vi "NI VeriStand - Get Custom Device Driver.vi"(8 "error in (no error)":errorcluster, 11 "Device Ref in":T4 format="%.0x") -> (0 "error out":errorcluster, 1 "Driver VI Path (Host)":T1, 2 "Driver VI Path (RT)":path, 3 "Device Ref out":T4 format="%.0x", 5 "Executon mode":T3)   [LabVIEW 2020, in "Custom Device Offline API.lvlib"]
uses:
  <vilib>/NI VeriStand/Custom Device Offline API/Custom Device Offline API.lvlib
  <vilib>/NI VeriStand/Custom Device API/Custom Device Item Ref.ctl
  <vilib>/NI VeriStand/Custom Device API/Custom Device Execution Mode.ctl
  <vilib>/NI VeriStand/Custom Device API/Path Specification.ctl
  <vilib>/NI VeriStand/Custom Device API/Path Type.ctl
  NationalInstruments.VeriStand.SystemDefinitionAPI
  <vilib>/NI VeriStand/Custom Device API/Custom Device API.lvlib
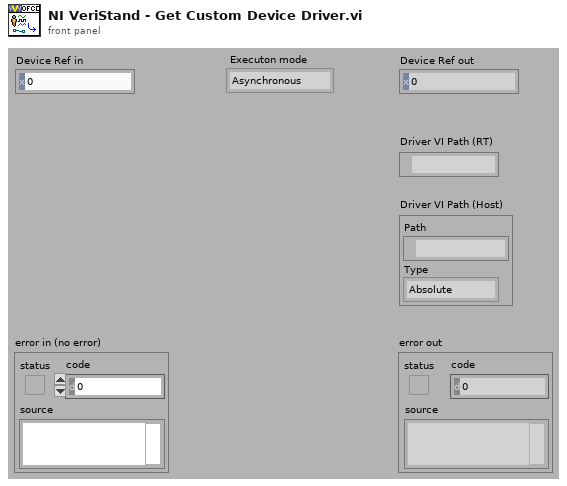
[diagram p1: front panel]
types:
  T1 = typedef "Custom Device API.lvlib/Path Specification.ctl" = cluster{"Path":path, "Type":T2}
  T2 = typedef "Custom Device API.lvlib/Path Type.ctl" = enum16{"Absolute", "To Base", "To Common Data Dir", "To Application Data Dir"}
  T3 = typedef "Custom Device API.lvlib/Custom Device Execution Mode.ctl" = enum16{"Asynchronous", "Inline HW Interface", "Inline Model Interface", "Inline Timing and Sync", "Asynchronous Timing and Sync"}
  T4 = typedef "Custom Device API.lvlib/Custom Device Item Ref.ctl" = u64
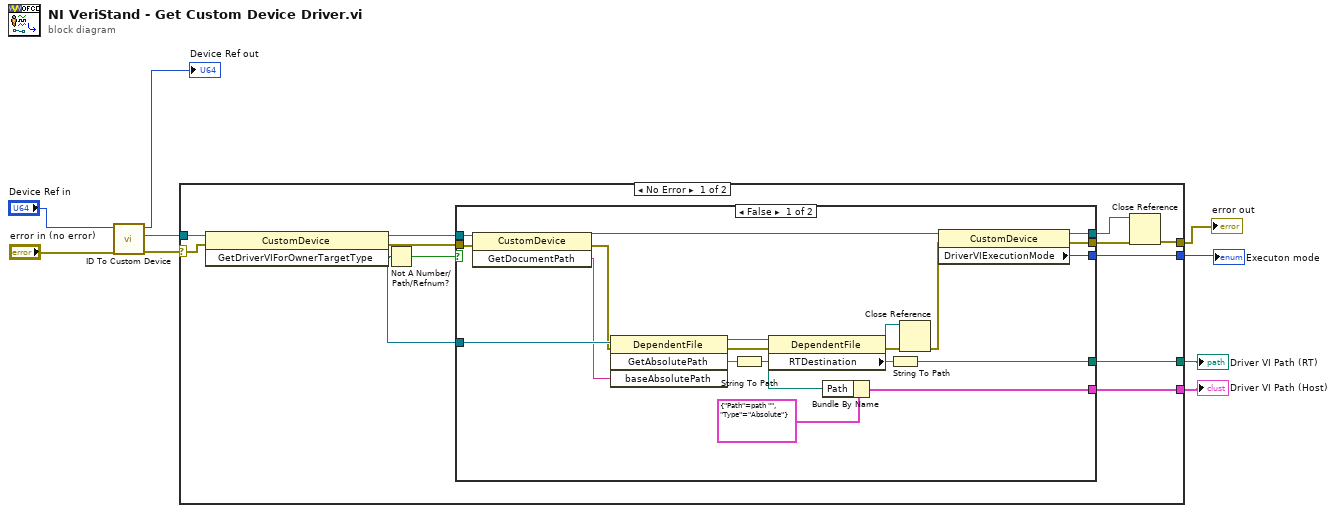
[diagram p0: block diagram]
diagram:
  n1 = call <vilib>:"ID To Custom Device.vi"("error in (no error)"="error in (no error)", "ID in"="Device Ref in") -> ("error out"=w7:errorcluster, "Device"=w5:refnum<k24>, "ID out"=→"Device Ref out":u64)  [unwired: 7 in]
  n2 = case shown="No Error" w7 {
    selector: w7 -> [w20 w44]
    tunnel: w5 -> [w21 _]
    tunnel: [w17 _] -> w4
    tunnel: [w13 w44] -> w3
    tunnel: [w11 _] -> w2
    tunnel: [w10 _] -> w1
    frame No Error {
      n3 = invoke class="CustomDevice" method="GetDriverVIForOwnerTargetType"(reference=w21, error in=w20) -> (reference out=w19:refnum<k24>, error out=w18:errorcluster, "GetDriverVIForOwnerTargetType"=w12:refnum<k24>)  [unwired: 1 in]
      n4 = Not A Number/Path/Refnum?(number/path/refnum=w12) -> (NaN/Path/Refnum?=w16:bool)
      n5 = case shown="False" w16 {
        tunnel: w19 -> [w35 w43]
        tunnel: w18 -> [w34 w42]
        tunnel: [w41 _] -> w17
        tunnel: [w40 w42] -> w15
        tunnel: [w39 w43] -> w14
        tunnel: w12 -> [w33 _]
        tunnel: [w24 _] -> w11
        tunnel: [w23 _] -> w10
        frame False {
          n6 = invoke class="CustomDevice" method="GetDocumentPath"(reference=w35, error in=w34) -> (reference out=w28:refnum<k24>, error out=w32:errorcluster, "GetDocumentPath"=w31:string)  [unwired: 1 in]
          n7 = invoke class="DependentFile" method="GetAbsolutePath"(reference=w33, error in=w32, "baseAbsolutePath"=w31) -> (reference out=w29:refnum<k24>, error out=w30:errorcluster, "GetAbsolutePath"=w27:string)  [unwired: 1 in, 1 out]
          n8 = String To Path(string=w27) -> (path=w26:path)
          n9 = property class="DependentFile"(reference=w29, error in=w30) -> (reference out=w37:refnum<k24>, error out=w38:errorcluster, "RTDestination"=w25:string)
          n10 = Bundle By Name(cluster=T1 {"Path"=path "", "Type"=enum."Absolute"} ("Driver VI Path (Host)"), "Path"=w26) -> (w23:T1)
          n11 = String To Path(string=w25) -> (path=w24:path)
          n12 = Close Reference(reference=w37, error in (no error)=w38) -> (error out=w36:errorcluster)
          n13 = property class="CustomDevice"(reference=w28, error in=w36) -> (reference out=w39:refnum<k24>, error out=w40:errorcluster, "DriverVIExecutionMode"=w41:u32)
        }
        frame True {
        }
      }
      n14 = Close Reference(reference=w14, error in (no error)=w15) -> (error out=w13:errorcluster)
    }
    frame Error {
    }
  }
  "error out" <- w3
  "Driver VI Path (RT)" <- w2
  "Executon mode" <- w4
  "Driver VI Path (Host)" <- w1
